vi "Load Image (Memory).vi"(8 "error in (no error)":errorcluster, 11 "Encoded Image":u8[](array[numeric])) -> (0 "error out":errorcluster, 2 "Image":T1)   [LabVIEW 2020, in "G-Image.lvlib"]
doc: "Load an image file from a byte array and return it as a LabVIEW picture.\n\nSupported image types:\nPNG, JPEG, BMP, GIF, TGA, PSD, HDR, PIC, PNM, QOI\n\nWhen loading an animated GIF, only the first frame will be returned. Use <b>Load Animated GIF Image.vi</b> to read all frames."
uses:
  G-Image.lvlib
  <vilib>/picture/picture.llb/imagedata.ctl
  Private/Get Image Data Size.vi
  <vilib>/picture/picture.llb/Create Mask By Alpha.vi
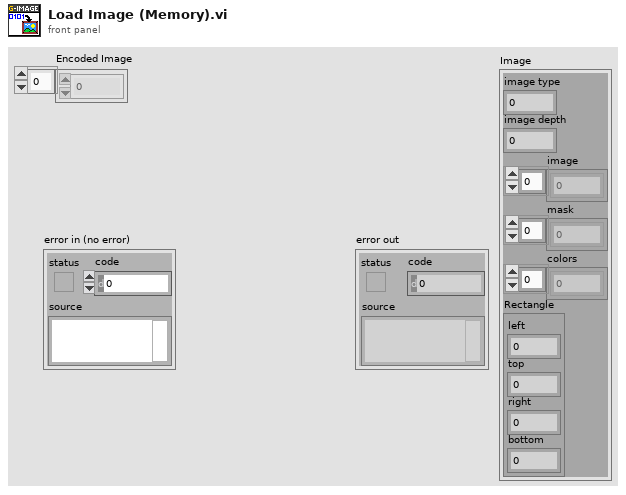
[diagram p1: front panel]
types:
  T1 = typedef "imagedata.ctl" = cluster{"image type":i32, "image depth":i32, "image":u8[], "mask":u8[], "colors":u32[], "Rectangle":cluster{"left":i16, "top":i16, "right":i16, "bottom":i16}}
  T2 = typedef "G-Image.lvlib/Extended Image.ctl" = cluster{"Image":T1, "Layers":i32, "Delays":i32[]}
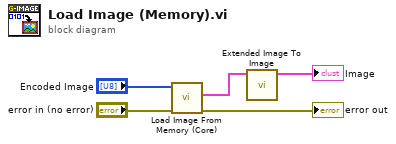
[diagram p0: block diagram]
diagram:
  n1 = call "Load Image From Memory (Core).vi"("error in (no error)"="error in (no error)", "Encoded Image"="Encoded Image") -> ("error out"=→"error out":errorcluster, "Extended Image"=w2:T2)  [unwired: 8 in]
  n2 = call "Extended Image To Image.vi"("Extended Image"=w2) -> ("Image"=→"Image":T1)  [unwired: 10 in]
